vi "Steering Motor Controler.vi"   [LabVIEW 2009]
uses:
  Motor Output Global.vi
  Motor Encoder Global.vi
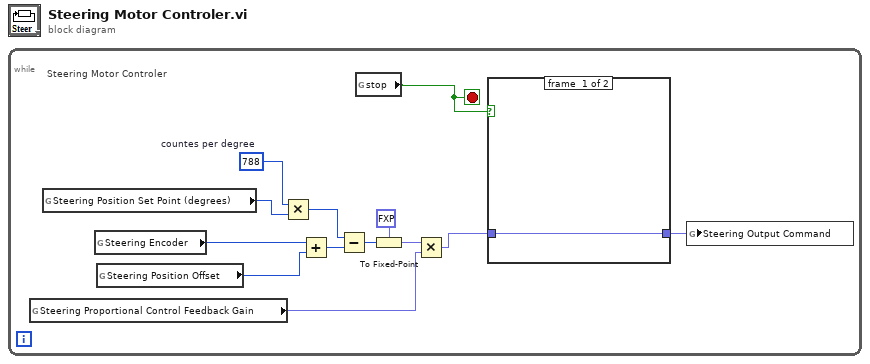
[diagram p0: block diagram]
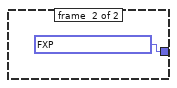
[diagram p2: hidden frame]
diagram:
  n1 = while {
    stop <- w6 stop-if-true
    w4 = 788  # countes per degree
    # "Steering Motor Controler"
    n2 = global read "Motor Encoder Global.vi" "Steering Proportional Control Feedback Gain"() -> (w5:fxp<+/-,20,5>)
    n3 = global read "Motor Encoder Global.vi" "Steering Position Set Point (degrees)"() -> (w1:i32)
    n4 = global read "Motor Encoder Global.vi" "Steering Encoder"() -> (w9:i32)
    n5 = global read "Motor Encoder Global.vi" "Steering Position Offset"() -> (w3:i32)
    n6 = Multiply(x=w4, y=w1) -> (x*y=w2:i32)
    n7 = Add(x=w9, y=w3) -> (x+y=w13:i32)
    n8 = Subtract(x=w2, y=w13) -> (x-y=w8:i32)
    n9 = global read "Motor Encoder Global.vi" "stop"() -> (w6:bool)
    n10 = To Fixed-Point(fixed-point type=fxp<+/-,20,5> 0.0, number=w8) -> (fixed-point=w7:fxp<+/-,20,5>)
    n11 = Multiply(x=w7, y=w5) -> (x*y=w11:fxp<+/-,20,5>)
    n12 = case shown="False" w6 {
      tunnel: w11 -> [w14 _]
      tunnel: [w14 fxp<+/-,20,5> 0.0] -> w10
      frame #0 {
      }
      frame #1 {
      }
    }
    n13 = global write "Motor Output Global.vi" "Steering Output Command"(w10) -> ()
  }
